vi "Main.vi"() -> ()   [LabVIEW 2019]
uses:
  <vilib>/myRIO/Instrument Drivers/Utilities/Utilities.lvlib
  WSCbot_V3_Toolkit.lvlibp
panel:
  out "error out 2":errorcluster
  in  "error in":errorcluster
  out "error out":errorcluster
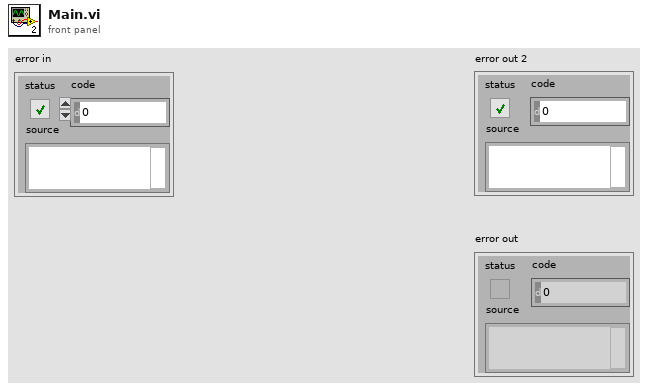
[diagram p1: front panel]
types:
  T1 = cluster{"Vmax (deg/s)":dbl, "acc (deg/sec^2)":dbl}
  T2 = cluster{"Direction":enum16{"Forward", "Tilt(R)", "Turn(CW)"}, "Target (cm||deg)":dbl}
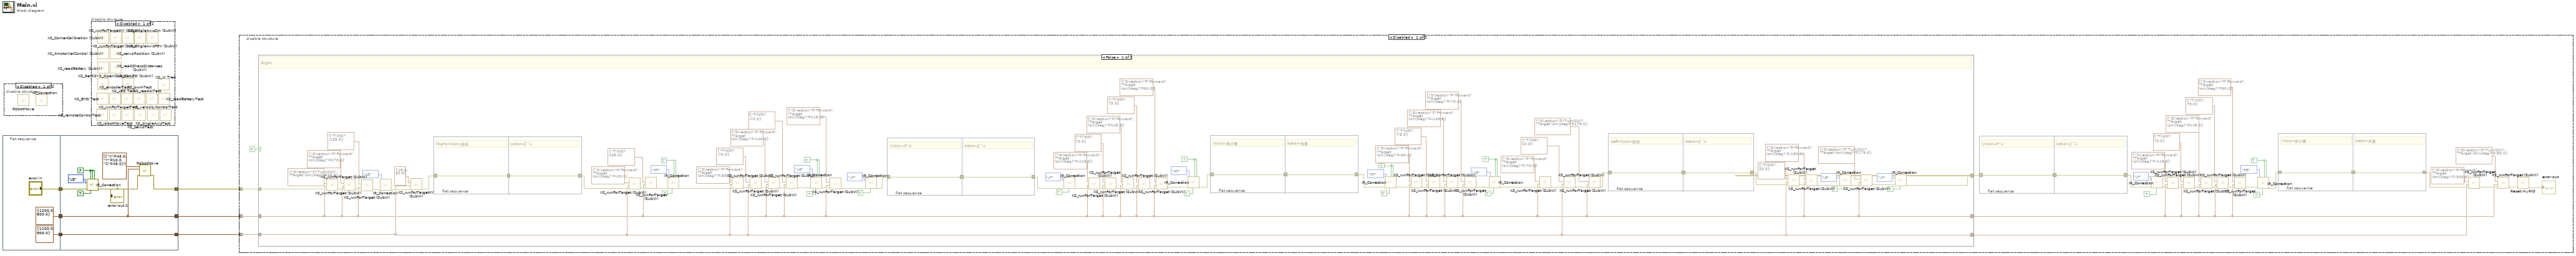
[diagram p0: block diagram]
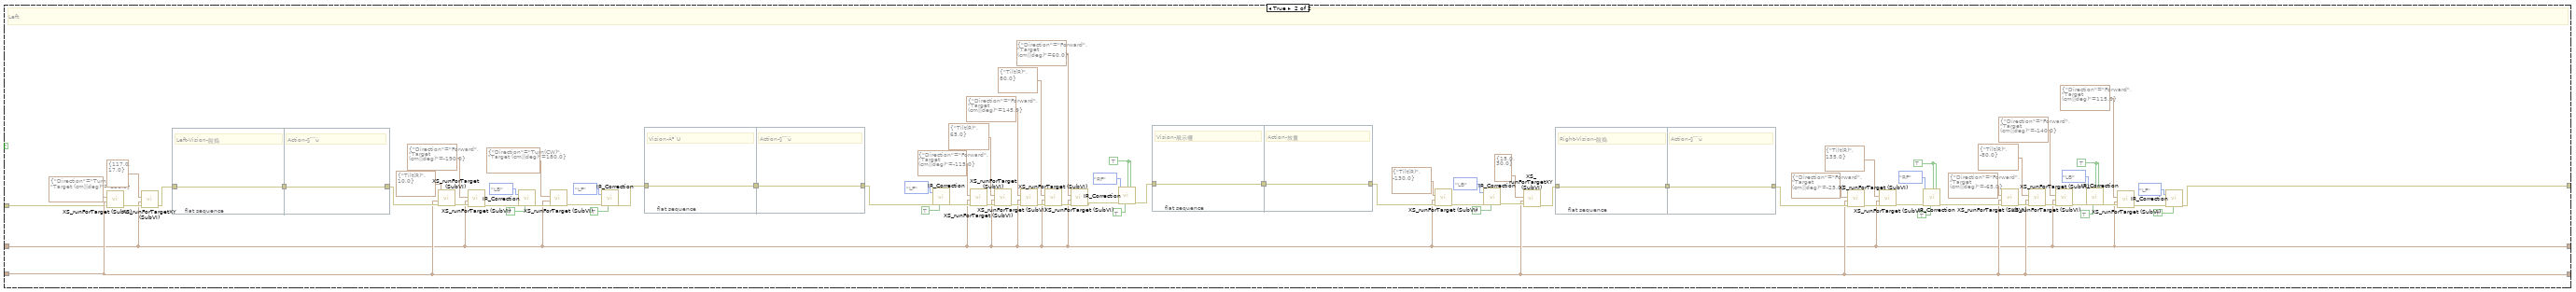
[diagram p3: hidden frame]
diagram:
  n1 = flat-sequence {
    tunnel: [T1 {"Vmax (deg/s)"=1100.0, "acc (deg/sec^2)"=900.0} ("Vmax&Acc")] -> w5
    tunnel: [T1 {"Vmax (deg/s)"=1200.0, "acc (deg/sec^2)"=800.0} ("Vmax&Acc")] -> w4
    tunnel: ["error in"] -> w1
    tunnel: w5 -> [w18]
    tunnel: w4 -> [w15]
    tunnel: [w18] -> w3
    tunnel: [w15] -> w6
    tunnel: [w16] -> w2
    tunnel: w1 -> [w17]
    frame #0 {
    }
    frame #1 {
      w11 = FALSE ("X Rate")
      n2 = call "IR_Correction.vi"("X Rate"=w11, "X_Rotate Rate"=w11, "Y Rate"=w11, "Mode"=enum16{"LF", "LB", "RF", "RB"}."LB", "error in"=w17, "width"=TRUE) -> ("error out"=w13:errorcluster)  [unwired: 9 in]
      "error out 2" <- w13
      n3 = call "RobotMove.vi"("error in (no error)"=w13, "Speed/ACC"=w15, "XYZ"=cluster{"X":dbl, "Y":dbl, "Z":dbl}[] [{"X"=45.0, "Y"=10.0, "Z"=45.0}]) -> ("error out"=w16:errorcluster)  [unwired: 8 in]
    }
  }
  n4 = disable-structure shown="Disabled" {
    frame Disabled {
      n5 = call "RobotMove.vi"() -> ()  [unwired: 11 in, 1 out]
      n6 = call "IR_Correction.vi"() -> ()  [unwired: 15 in, 1 out]
    }
    frame Enabled {
    }
  }
  n7 = disable-structure shown="Disabled" {
    frame Disabled {
      n8 = call <vilib>:"XS_remoteControlTest.vi"() -> ()  [unwired: 12 in]
      n9 = call <vilib>:"XS_EMS Test.vi"() -> ()  [unwired: 12 in]
      n10 = call <vilib>:"XS_ReMiSYS_Open(SubVI).vi"() -> ()  [unwired: 10 in, 2 out]
      n11 = call <vilib>:"XS_CornerCalibration (SubVI).vi"() -> ()  [unwired: 11 in, 1 out]
      n12 = call <vilib>:"XS_4motorVelControl (SubVI).vi"() -> ()  [unwired: 9 in, 3 out]
      n13 = call <vilib>:"XS_readBattery (SubVI).vi"() -> ()  [unwired: 10 in, 2 out]
      n14 = call <vilib>:"XS_encoderTest.vi"() -> ()  [unwired: 12 in]
      n15 = call <vilib>:"XS_robotMoveTest.vi"() -> ()  [unwired: 12 in]
      n16 = call <vilib>:"XS_runForTarget (SubVI).vi"() -> ()  [unwired: 11 in, 1 out]
      n17 = call <vilib>:"XS_servoPosition (SubVI).vi"() -> ()  [unwired: 11 in, 1 out]
      n18 = call <vilib>:"XS_readSharpDistances (SubVI).vi"() -> ()  [unwired: 9 in, 3 out]
      n19 = call <vilib>:"XS_LED Test.vi"() -> ()  [unwired: 12 in]
      n20 = call <vilib>:"XS_runForTargetTest.vi"() -> ()  [unwired: 12 in]
      n21 = call <vilib>:"XS_runForTargetXY (SubVI).vi"() -> ()  [unwired: 11 in, 1 out]
      n22 = call <vilib>:"XS_SetLED (SubVI).vi"() -> ()  [unwired: 11 in, 1 out]
      n23 = call <vilib>:"XS_pwmTest.vi"() -> ()  [unwired: 12 in]
      n24 = call <vilib>:"XS_singleAxisCm (SubVI).vi"() -> ()  [unwired: 10 in, 2 out]
      n25 = call <vilib>:"XS_servoTest.vi"() -> ()  [unwired: 12 in]
      n26 = call <vilib>:"XS_readAITest.vi"() -> ()  [unwired: 12 in]
      n27 = call <vilib>:"XS_singleAxisFGV (SubVI).vi"() -> ()  [unwired: 9 in, 3 out]
      n28 = call <vilib>:"XS_singleAxisTest.vi"() -> ()  [unwired: 12 in]
      n29 = call <vilib>:"XS_VI Tree.vi"() -> ()  [unwired: 12 in]
      n30 = call <vilib>:"XS_readBatteryTest.vi"() -> ()  [unwired: 12 in]
      n31 = call <vilib>:"XS_velocityControlTest.vi"() -> ()  [unwired: 12 in]
    }
    frame Enabled {
    }
  }
  n32 = disable-structure shown="Disabled" {
    disable-tunnel: w6 -> [w49 _]
    disable-tunnel: w3 -> [w35 _]
    disable-tunnel: w2 -> [w25 _]
    frame Disabled {
      w30 = TRUE ("Y Rate Control")
      n33 = case shown="False" FALSE {
        tunnel: w49 -> [w56 w161]
        tunnel: w35 -> [w63 w163]
        tunnel: [w64 w169] -> w33
        tunnel: [w63 w163] -> w26
        tunnel: [w56 w161] -> w21
        tunnel: w25 -> [w138 w162]
        frame False {
          w83 = TRUE ("Y Rate Control")
          w87 = TRUE ("Y Rate Control")
          w96 = TRUE ("Y Rate Control")
          w120 = TRUE ("Y Rate Control")
          w126 = TRUE ("Y Rate Control")
          # "Right"
          n34 = call <vilib>:"XS_runForTarget (SubVI).vi"("error in (no error)"=w138, "Vmax&Acc"=w56, "Dir&Target"=T2 {"Direction"=enum."Turn(CW)", "Target (cm||deg)"=46.0}) -> ("error out"=w148:errorcluster)  [unwired: 8 in]
          n35 = call <vilib>:"XS_runForTarget (SubVI).vi"("error in (no error)"=w148, "Vmax&Acc"=w56, "Dir&Target"=T2 {"Direction"=enum."Forward", "Target (cm||deg)"=270.0}) -> ("error out"=w147:errorcluster)  [unwired: 8 in]
          n36 = call <vilib>:"XS_runForTarget (SubVI).vi"("error in (no error)"=w147, "Vmax&Acc"=w56, "Dir&Target"=T2 {"Direction"=enum."Tilt(R)", "Target (cm||deg)"=-135.0}) -> ("error out"=w146:errorcluster)  [unwired: 8 in]
          n37 = call "IR_Correction.vi"("Mode"=enum16{"LF", "LB", "RF", "RB"}."LB", "error in"=w146) -> ("error out"=w145:errorcluster)  [unwired: 17 in]
          n38 = call <vilib>:"XS_runForTargetXY (SubVI).vi"("error in (no error)"=w145, "Vmax&Acc"=w63, "Target"=cluster{"X":dbl, "Y":dbl} {"X"=15.0, "Y"=30.0}) -> ("error out"=w114:errorcluster)  [unwired: 8 in]
          n39 = flat-sequence {
            tunnel: w114 -> [w159]
            tunnel: [w159] -> w137
            tunnel: [w160] -> w123
            tunnel: w137 -> [w160]
            frame #0 {
              # "Right-Vision-脸捣"
            }
            frame #1 {
              # "Action-§¨¨ú"
            }
          }
          n40 = call <vilib>:"XS_runForTarget (SubVI).vi"("error in (no error)"=w123, "Vmax&Acc"=w63, "Dir&Target"=T2 {"Direction"=enum."Forward", "Target (cm||deg)"=-20.0}) -> ("error out"=w135:errorcluster)  [unwired: 8 in]
          n41 = call <vilib>:"XS_runForTarget (SubVI).vi"("error in (no error)"=w135, "Vmax&Acc"=w56, "Dir&Target"=T2 {"Direction"=enum."Tilt(R)", "Target (cm||deg)"=135.0}) -> ("error out"=w119:errorcluster)  [unwired: 8 in]
          n42 = call "IR_Correction.vi"("Mode"=enum16{"LF", "LB", "RF", "RB"}."RF", "error in"=w119, "width"=TRUE, "Y Rate Control"=w120, "Rotate Rate Control"=w120) -> ("error out"=w118:errorcluster)  [unwired: 14 in]
          n43 = call <vilib>:"XS_runForTarget (SubVI).vi"("error in (no error)"=w118, "Vmax&Acc"=w63, "Dir&Target"=T2 {"Direction"=enum."Forward", "Target (cm||deg)"=-65.0}) -> ("error out"=w132:errorcluster)  [unwired: 8 in]
          n44 = call <vilib>:"XS_runForTarget (SubVI).vi"("error in (no error)"=w132, "Vmax&Acc"=w63, "Dir&Target"=T2 {"Direction"=enum."Tilt(R)", "Target (cm||deg)"=-70.0}) -> ("error out"=w130:errorcluster)  [unwired: 8 in]
          n45 = call <vilib>:"XS_runForTarget (SubVI).vi"("error in (no error)"=w130, "Vmax&Acc"=w56, "Dir&Target"=T2 {"Direction"=enum."Forward", "Target (cm||deg)"=-140.0}) -> ("error out"=w62:errorcluster)  [unwired: 8 in]
          n46 = call <vilib>:"XS_runForTarget (SubVI).vi"("error in (no error)"=w62, "Vmax&Acc"=w56, "Dir&Target"=T2 {"Direction"=enum."Tilt(R)", "Target (cm||deg)"=-70.0}) -> ("error out"=w61:errorcluster)  [unwired: 8 in]
          n47 = call "IR_Correction.vi"("Mode"=enum16{"LF", "LB", "RF", "RB"}."LB", "error in"=w61, "width"=TRUE, "Y Rate Control"=w126, "Rotate Rate Control"=w126) -> ("error out"=w125:errorcluster)  [unwired: 14 in]
          n48 = call <vilib>:"XS_runForTarget (SubVI).vi"("error in (no error)"=w125, "Vmax&Acc"=w56, "Dir&Target"=T2 {"Direction"=enum."Forward", "Target (cm||deg)"=115.0}) -> ("error out"=w115:errorcluster)  [unwired: 8 in]
          n49 = call "IR_Correction.vi"("Mode"=enum16{"LF", "LB", "RF", "RB"}."LF", "error in"=w115, "width"=TRUE) -> ("error out"=w94:errorcluster)  [unwired: 16 in]
          n50 = flat-sequence {
            tunnel: w94 -> [w157]
            tunnel: [w157] -> w113
            tunnel: [w158] -> w99
            tunnel: w113 -> [w158]
            frame #0 {
              # "Vision-Á³´U"
            }
            frame #1 {
              # "Action-§¨¨ú"
            }
          }
          n51 = call "IR_Correction.vi"("Mode"=enum16{"LF", "LB", "RF", "RB"}."LF", "error in"=w99, "width"=TRUE) -> ("error out"=w107:errorcluster)  [unwired: 16 in]
          n52 = call <vilib>:"XS_runForTarget (SubVI).vi"("error in (no error)"=w107, "Vmax&Acc"=w56, "Dir&Target"=T2 {"Direction"=enum."Forward", "Target (cm||deg)"=-115.0}) -> ("error out"=w109:errorcluster)  [unwired: 8 in]
          n53 = call <vilib>:"XS_runForTarget (SubVI).vi"("error in (no error)"=w109, "Vmax&Acc"=w56, "Dir&Target"=T2 {"Direction"=enum."Tilt(R)", "Target (cm||deg)"=70.0}) -> ("error out"=w106:errorcluster)  [unwired: 8 in]
          n54 = call <vilib>:"XS_runForTarget (SubVI).vi"("error in (no error)"=w106, "Vmax&Acc"=w56, "Dir&Target"=T2 {"Direction"=enum."Forward", "Target (cm||deg)"=145.0}) -> ("error out"=w102:errorcluster)  [unwired: 8 in]
          n55 = call <vilib>:"XS_runForTarget (SubVI).vi"("error in (no error)"=w102, "Vmax&Acc"=w56, "Dir&Target"=T2 {"Direction"=enum."Tilt(R)", "Target (cm||deg)"=75.0}) -> ("error out"=w101:errorcluster)  [unwired: 8 in]
          n56 = call <vilib>:"XS_runForTarget (SubVI).vi"("error in (no error)"=w101, "Vmax&Acc"=w56, "Dir&Target"=T2 {"Direction"=enum."Forward", "Target (cm||deg)"=60.0}) -> ("error out"=w95:errorcluster)  [unwired: 8 in]
          n57 = call "IR_Correction.vi"("Mode"=enum16{"LF", "LB", "RF", "RB"}."RF", "error in"=w95, "width"=TRUE, "Y Rate Control"=w96, "Rotate Rate Control"=w96) -> ("error out"=w81:errorcluster)  [unwired: 14 in]
          n58 = flat-sequence {
            tunnel: w81 -> [w155]
            tunnel: [w155] -> w112
            tunnel: [w156] -> w80
            tunnel: w112 -> [w156]
            frame #0 {
              # "Vision-展示櫃"
            }
            frame #1 {
              # "Action-放置"
            }
          }
          n59 = call "IR_Correction.vi"("Mode"=enum16{"LF", "LB", "RF", "RB"}."RF", "error in"=w80, "width"=TRUE, "Y Rate Control"=w83, "Rotate Rate Control"=w83) -> ("error out"=w82:errorcluster)  [unwired: 14 in]
          n60 = call <vilib>:"XS_runForTarget (SubVI).vi"("error in (no error)"=w82, "Vmax&Acc"=w56, "Dir&Target"=T2 {"Direction"=enum."Forward", "Target (cm||deg)"=-60.0}) -> ("error out"=w92:errorcluster)  [unwired: 8 in]
          n61 = call <vilib>:"XS_runForTarget (SubVI).vi"("error in (no error)"=w92, "Vmax&Acc"=w56, "Dir&Target"=T2 {"Direction"=enum."Tilt(R)", "Target (cm||deg)"=-75.0}) -> ("error out"=w90:errorcluster)  [unwired: 8 in]
          n62 = call <vilib>:"XS_runForTarget (SubVI).vi"("error in (no error)"=w90, "Vmax&Acc"=w56, "Dir&Target"=T2 {"Direction"=enum."Forward", "Target (cm||deg)"=-145.0}) -> ("error out"=w59:errorcluster)  [unwired: 8 in]
          n63 = call <vilib>:"XS_runForTarget (SubVI).vi"("error in (no error)"=w59, "Vmax&Acc"=w56, "Dir&Target"=T2 {"Direction"=enum."Forward", "Target (cm||deg)"=-70.0}) -> ("error out"=w58:errorcluster)  [unwired: 8 in]
          n64 = call "IR_Correction.vi"("Mode"=enum16{"LF", "LB", "RF", "RB"}."LB", "error in"=w58, "width"=TRUE, "Y Rate Control"=w87, "Rotate Rate Control"=w87) -> ("error out"=w79:errorcluster)  [unwired: 14 in]
          n65 = call <vilib>:"XS_runForTarget (SubVI).vi"("error in (no error)"=w79, "Vmax&Acc"=w56, "Dir&Target"=T2 {"Direction"=enum."Forward", "Target (cm||deg)"=-70.0}) -> ("error out"=w142:errorcluster)  [unwired: 8 in]
          n66 = call <vilib>:"XS_runForTarget (SubVI).vi"("error in (no error)"=w142, "Vmax&Acc"=w63, "Dir&Target"=T2 {"Direction"=enum."Tilt(R)", "Target (cm||deg)"=10.0}) -> ("error out"=w141:errorcluster)  [unwired: 8 in]
          n67 = call <vilib>:"XS_runForTarget (SubVI).vi"("error in (no error)"=w141, "Vmax&Acc"=w56, "Dir&Target"=T2 {"Direction"=enum."Turn(CW)", "Target (cm||deg)"=179.0}) -> ("error out"=w65:errorcluster)  [unwired: 8 in]
          n68 = flat-sequence {
            tunnel: w65 -> [w153]
            tunnel: [w153] -> w78
            tunnel: [w154] -> w76
            tunnel: w78 -> [w154]
            frame #0 {
              # "Left-Vision-脸捣"
            }
            frame #1 {
              # "Action-§¨¨ú"
            }
          }
          n69 = call <vilib>:"XS_runForTarget (SubVI).vi"("error in (no error)"=w76, "Vmax&Acc"=w63, "Dir&Target"=T2 {"Direction"=enum."Tilt(R)", "Target (cm||deg)"=20.0}) -> ("error out"=w73:errorcluster)  [unwired: 8 in]
          n70 = call <vilib>:"XS_runForTarget (SubVI).vi"("error in (no error)"=w73, "Vmax&Acc"=w56, "Dir&Target"=T2 {"Direction"=enum."Forward", "Target (cm||deg)"=-190.0}) -> ("error out"=w74:errorcluster)  [unwired: 8 in]
          n71 = call "IR_Correction.vi"("Mode"=enum16{"LF", "LB", "RF", "RB"}."LB", "error in"=w74, "width"=TRUE) -> ("error out"=w75:errorcluster)  [unwired: 16 in]
          n72 = call <vilib>:"XS_runForTarget (SubVI).vi"("error in (no error)"=w75, "Vmax&Acc"=w56, "Dir&Target"=T2 {"Direction"=enum."Turn(CW)", "Target (cm||deg)"=179.0}) -> ("error out"=w77:errorcluster)  [unwired: 8 in]
          n73 = call "IR_Correction.vi"("Mode"=enum16{"LF", "LB", "RF", "RB"}."LF", "error in"=w77, "width"=TRUE) -> ("error out"=w64:errorcluster)  [unwired: 16 in]
        }
        frame True {
          w166 = TRUE ("Y Rate Control")
          w175 = TRUE ("Y Rate Control")
          w200 = TRUE ("Y Rate Control")
          # "Left"
          n74 = call <vilib>:"XS_runForTarget (SubVI).vi"("error in (no error)"=w162, "Vmax&Acc"=w163, "Dir&Target"=T2 {"Direction"=enum."Turn(CW)", "Target (cm||deg)"=-136.0}) -> ("error out"=w190:errorcluster)  [unwired: 8 in]
          n75 = call <vilib>:"XS_runForTargetXY (SubVI).vi"("error in (no error)"=w190, "Vmax&Acc"=w161, "Target"=cluster{"X":dbl, "Y":dbl} {"X"=117.0, "Y"=17.0}) -> ("error out"=w187:errorcluster)  [unwired: 8 in]
          n76 = flat-sequence {
            tunnel: w187 -> [w241]
            tunnel: [w241] -> w234
            tunnel: [w242] -> w186
            tunnel: w234 -> [w242]
            frame #0 {
              # "Left-Vision-脸捣"
            }
            frame #1 {
              # "Action-§¨¨ú"
            }
          }
          n77 = call <vilib>:"XS_runForTarget (SubVI).vi"("error in (no error)"=w186, "Vmax&Acc"=w163, "Dir&Target"=T2 {"Direction"=enum."Tilt(R)", "Target (cm||deg)"=10.0}) -> ("error out"=w228:errorcluster)  [unwired: 8 in]
          n78 = call <vilib>:"XS_runForTarget (SubVI).vi"("error in (no error)"=w228, "Vmax&Acc"=w161, "Dir&Target"=T2 {"Direction"=enum."Forward", "Target (cm||deg)"=-190.0}) -> ("error out"=w192:errorcluster)  [unwired: 8 in]
          n79 = call "IR_Correction.vi"("Mode"=enum16{"LF", "LB", "RF", "RB"}."LB", "error in"=w192, "width"=TRUE) -> ("error out"=w191:errorcluster)  [unwired: 16 in]
          n80 = call <vilib>:"XS_runForTarget (SubVI).vi"("error in (no error)"=w191, "Vmax&Acc"=w161, "Dir&Target"=T2 {"Direction"=enum."Turn(CW)", "Target (cm||deg)"=180.0}) -> ("error out"=w182:errorcluster)  [unwired: 8 in]
          n81 = call "IR_Correction.vi"("Mode"=enum16{"LF", "LB", "RF", "RB"}."LF", "error in"=w182, "width"=TRUE) -> ("error out"=w181:errorcluster)  [unwired: 16 in]
          n82 = flat-sequence {
            tunnel: w181 -> [w239]
            tunnel: [w239] -> w233
            tunnel: [w240] -> w185
            tunnel: w233 -> [w240]
            frame #0 {
              # "Vision-Á³´U"
            }
            frame #1 {
              # "Action-§¨¨ú"
            }
          }
          n83 = call "IR_Correction.vi"("Mode"=enum16{"LF", "LB", "RF", "RB"}."LF", "error in"=w185, "width"=TRUE) -> ("error out"=w209:errorcluster)  [unwired: 16 in]
          n84 = call <vilib>:"XS_runForTarget (SubVI).vi"("error in (no error)"=w209, "Vmax&Acc"=w161, "Dir&Target"=T2 {"Direction"=enum."Forward", "Target (cm||deg)"=-115.0}) -> ("error out"=w211:errorcluster)  [unwired: 8 in]
          n85 = call <vilib>:"XS_runForTarget (SubVI).vi"("error in (no error)"=w211, "Vmax&Acc"=w161, "Dir&Target"=T2 {"Direction"=enum."Tilt(R)", "Target (cm||deg)"=65.0}) -> ("error out"=w208:errorcluster)  [unwired: 8 in]
          n86 = call <vilib>:"XS_runForTarget (SubVI).vi"("error in (no error)"=w208, "Vmax&Acc"=w161, "Dir&Target"=T2 {"Direction"=enum."Forward", "Target (cm||deg)"=145.0}) -> ("error out"=w204:errorcluster)  [unwired: 8 in]
          n87 = call <vilib>:"XS_runForTarget (SubVI).vi"("error in (no error)"=w204, "Vmax&Acc"=w161, "Dir&Target"=T2 {"Direction"=enum."Tilt(R)", "Target (cm||deg)"=80.0}) -> ("error out"=w203:errorcluster)  [unwired: 8 in]
          n88 = call <vilib>:"XS_runForTarget (SubVI).vi"("error in (no error)"=w203, "Vmax&Acc"=w161, "Dir&Target"=T2 {"Direction"=enum."Forward", "Target (cm||deg)"=60.0}) -> ("error out"=w165:errorcluster)  [unwired: 8 in]
          n89 = call "IR_Correction.vi"("Mode"=enum16{"LF", "LB", "RF", "RB"}."RF", "error in"=w165, "width"=TRUE, "Y Rate Control"=w166, "Rotate Rate Control"=w166) -> ("error out"=w164:errorcluster)  [unwired: 14 in]
          n90 = flat-sequence {
            tunnel: w164 -> [w237]
            tunnel: [w237] -> w232
            tunnel: [w238] -> w180
            tunnel: w232 -> [w238]
            frame #0 {
              # "Vision-展示櫃"
            }
            frame #1 {
              # "Action-放置"
            }
          }
          n91 = call <vilib>:"XS_runForTarget (SubVI).vi"("error in (no error)"=w180, "Vmax&Acc"=w161, "Dir&Target"=T2 {"Direction"=enum."Tilt(R)", "Target (cm||deg)"=-130.0}) -> ("error out"=w215:errorcluster)  [unwired: 8 in]
          n92 = call "IR_Correction.vi"("Mode"=enum16{"LF", "LB", "RF", "RB"}."LB", "error in"=w215, "width"=FALSE) -> ("error out"=w214:errorcluster)  [unwired: 16 in]
          n93 = call <vilib>:"XS_runForTargetXY (SubVI).vi"("error in (no error)"=w214, "Vmax&Acc"=w163, "Target"=cluster{"X":dbl, "Y":dbl} {"X"=15.0, "Y"=30.0}) -> ("error out"=w179:errorcluster)  [unwired: 8 in]
          n94 = flat-sequence {
            tunnel: w179 -> [w235]
            tunnel: [w235] -> w231
            tunnel: [w236] -> w178
            tunnel: w231 -> [w236]
            frame #0 {
              # "Right-Vision-脸捣"
            }
            frame #1 {
              # "Action-§¨¨ú"
            }
          }
          n95 = call <vilib>:"XS_runForTarget (SubVI).vi"("error in (no error)"=w178, "Vmax&Acc"=w163, "Dir&Target"=T2 {"Direction"=enum."Forward", "Target (cm||deg)"=-25.0}) -> ("error out"=w224:errorcluster)  [unwired: 8 in]
          n96 = call <vilib>:"XS_runForTarget (SubVI).vi"("error in (no error)"=w224, "Vmax&Acc"=w161, "Dir&Target"=T2 {"Direction"=enum."Tilt(R)", "Target (cm||deg)"=135.0}) -> ("error out"=w174:errorcluster)  [unwired: 8 in]
          n97 = call "IR_Correction.vi"("Mode"=enum16{"LF", "LB", "RF", "RB"}."RF", "error in"=w174, "width"=TRUE, "Y Rate Control"=w175, "Rotate Rate Control"=w175) -> ("error out"=w173:errorcluster)  [unwired: 14 in]
          n98 = call <vilib>:"XS_runForTarget (SubVI).vi"("error in (no error)"=w173, "Vmax&Acc"=w163, "Dir&Target"=T2 {"Direction"=enum."Forward", "Target (cm||deg)"=-65.0}) -> ("error out"=w221:errorcluster)  [unwired: 8 in]
          n99 = call <vilib>:"XS_runForTarget (SubVI).vi"("error in (no error)"=w221, "Vmax&Acc"=w163, "Dir&Target"=T2 {"Direction"=enum."Tilt(R)", "Target (cm||deg)"=-80.0}) -> ("error out"=w219:errorcluster)  [unwired: 8 in]
          n100 = call <vilib>:"XS_runForTarget (SubVI).vi"("error in (no error)"=w219, "Vmax&Acc"=w161, "Dir&Target"=T2 {"Direction"=enum."Forward", "Target (cm||deg)"=-140.0}) -> ("error out"=w199:errorcluster)  [unwired: 8 in]
          n101 = call "IR_Correction.vi"("Mode"=enum16{"LF", "LB", "RF", "RB"}."LB", "error in"=w199, "width"=TRUE, "Y Rate Control"=w200, "Rotate Rate Control"=w200) -> ("error out"=w198:errorcluster)  [unwired: 14 in]
          n102 = call <vilib>:"XS_runForTarget (SubVI).vi"("error in (no error)"=w198, "Vmax&Acc"=w161, "Dir&Target"=T2 {"Direction"=enum."Forward", "Target (cm||deg)"=115.0}) -> ("error out"=w170:errorcluster)  [unwired: 8 in]
          n103 = call "IR_Correction.vi"("Mode"=enum16{"LF", "LB", "RF", "RB"}."LF", "error in"=w170, "width"=TRUE) -> ("error out"=w169:errorcluster)  [unwired: 16 in]
        }
      }
      n104 = flat-sequence {
        tunnel: w33 -> [w54]
        tunnel: [w54] -> w51
        tunnel: [w55] -> w32
        tunnel: w51 -> [w55]
        frame #0 {
          # "Vision-Á³´U"
        }
        frame #1 {
          # "Action-§¨¨ú"
        }
      }
      n105 = call "IR_Correction.vi"("Mode"=enum16{"LF", "LB", "RF", "RB"}."LF", "error in"=w32, "width"=TRUE) -> ("error out"=w44:errorcluster)  [unwired: 16 in]
      n106 = call <vilib>:"XS_runForTarget (SubVI).vi"("error in (no error)"=w44, "Vmax&Acc"=w21, "Dir&Target"=T2 {"Direction"=enum."Forward", "Target (cm||deg)"=-115.0}) -> ("error out"=w46:errorcluster)  [unwired: 8 in]
      n107 = call <vilib>:"XS_runForTarget (SubVI).vi"("error in (no error)"=w46, "Vmax&Acc"=w21, "Dir&Target"=T2 {"Direction"=enum."Tilt(R)", "Target (cm||deg)"=70.0}) -> ("error out"=w43:errorcluster)  [unwired: 8 in]
      n108 = call <vilib>:"XS_runForTarget (SubVI).vi"("error in (no error)"=w43, "Vmax&Acc"=w21, "Dir&Target"=T2 {"Direction"=enum."Forward", "Target (cm||deg)"=145.0}) -> ("error out"=w39:errorcluster)  [unwired: 8 in]
      n109 = call <vilib>:"XS_runForTarget (SubVI).vi"("error in (no error)"=w39, "Vmax&Acc"=w21, "Dir&Target"=T2 {"Direction"=enum."Tilt(R)", "Target (cm||deg)"=75.0}) -> ("error out"=w38:errorcluster)  [unwired: 8 in]
      n110 = call <vilib>:"XS_runForTarget (SubVI).vi"("error in (no error)"=w38, "Vmax&Acc"=w21, "Dir&Target"=T2 {"Direction"=enum."Forward", "Target (cm||deg)"=60.0}) -> ("error out"=w28:errorcluster)  [unwired: 8 in]
      n111 = call "IR_Correction.vi"("Mode"=enum16{"LF", "LB", "RF", "RB"}."RB", "error in"=w28, "width"=TRUE, "Y Rate Control"=w30, "Rotate Rate Control"=w30) -> ("error out"=w27:errorcluster)  [unwired: 14 in]
      n112 = flat-sequence {
        tunnel: w27 -> [w52]
        tunnel: [w52] -> w50
        tunnel: [w53] -> w34
        tunnel: w50 -> [w53]
        frame #0 {
          # "Vision-展示櫃"
        }
        frame #1 {
          # "Action-放置"
        }
      }
      n113 = call <vilib>:"XS_runForTarget (SubVI).vi"("error in (no error)"=w34, "Vmax&Acc"=w26, "Dir&Target"=T2 {"Direction"=enum."Forward", "Target (cm||deg)"=-300.0}) -> ("error out"=w23:errorcluster)  [unwired: 8 in]
      n114 = call <vilib>:"XS_runForTarget (SubVI).vi"("error in (no error)"=w23, "Vmax&Acc"=w21, "Dir&Target"=T2 {"Direction"=enum."Turn(CW)", "Target (cm||deg)"=-90.0}) -> ("error out"=w20:errorcluster)  [unwired: 8 in]
      n115 = call <vilib>:"Reset myRIO.vi"("error in (no error)"=w20) -> ("error out"=→"error out":errorcluster)  [unwired: 10 in]
    }
    frame Enabled {
    }
  }
